vi "DataTreeCtrl signalToSpecData.vi"(8 "error in (no error)":errorcluster, 10 "signalMultiData":waveform(sgl)[](array[waveform]), 11 "DataTreeCtrl in":refnum<class "DataTreeCtrl.lvclass">) -> (0 "error out":errorcluster, 1 "labelName":T2, 2 "scanSigInfo":T1(array[cluster]), 3 "DataTreeCtrl out":refnum<class "DataTreeCtrl.lvclass">, 4 "mergeValid?":bool, 5 "plotName":string[](array[string]))   [LabVIEW 2018, in "DataTreeCtrl.lvclass"]
uses:
  DataTreeCtrl.lvclass
  DataTreeCtrl.lvclass/DataTreeCtrl.ctl
  PublicSubVI/Overload/Experiment Condition/_PC_Pub_ExpCondiValue_Script.vi
  PublicSubVI/Class/Sig2MS/Sig2MS.lvclass
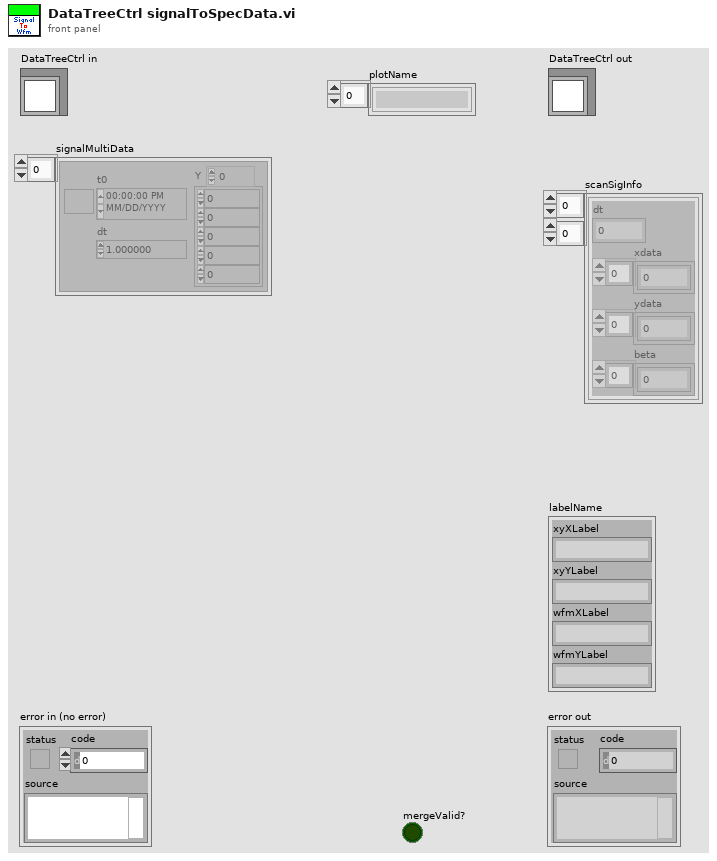
[diagram p1: front panel]
types:
  T1 = cluster{"dt":dbl, "xdata":dbl[], "ydata":sgl[], "beta":dbl[]}[][]
  T2 = cluster{"xyXLabel":string, "xyYLabel":string, "wfmXLabel":string, "wfmYLabel":string}
  T3 = enum16{"init", "loadScript", "newScript", "runScript", "close"}
  T4 = cluster{"startTime":dbl, "scanSig":cluster{"priDt":dbl, "priXData":dbl[], "priYData":sgl[], "beta":dbl[]}[], "ionSig":cluster{"secDt":dbl, "secYData":sgl[]}[]}
  T5 = cluster{"startTime":dbl, "scanData":cluster{"dt":dbl, "xdata":dbl[], "ydata":sgl[], "beta":dbl[]}[], "xyXLabel":string, "xyYLabel":string, "wfmXLabel":string, "wfmYLabel":string, "ionData":cluster{"dt":dbl, "ydata":sgl[]}[], "ionXLabel":string, "ionYLabel":string}
  T6 = cluster{"dt":dbl, "xdata":dbl[], "ydata":sgl[], "beta":dbl[]}[]
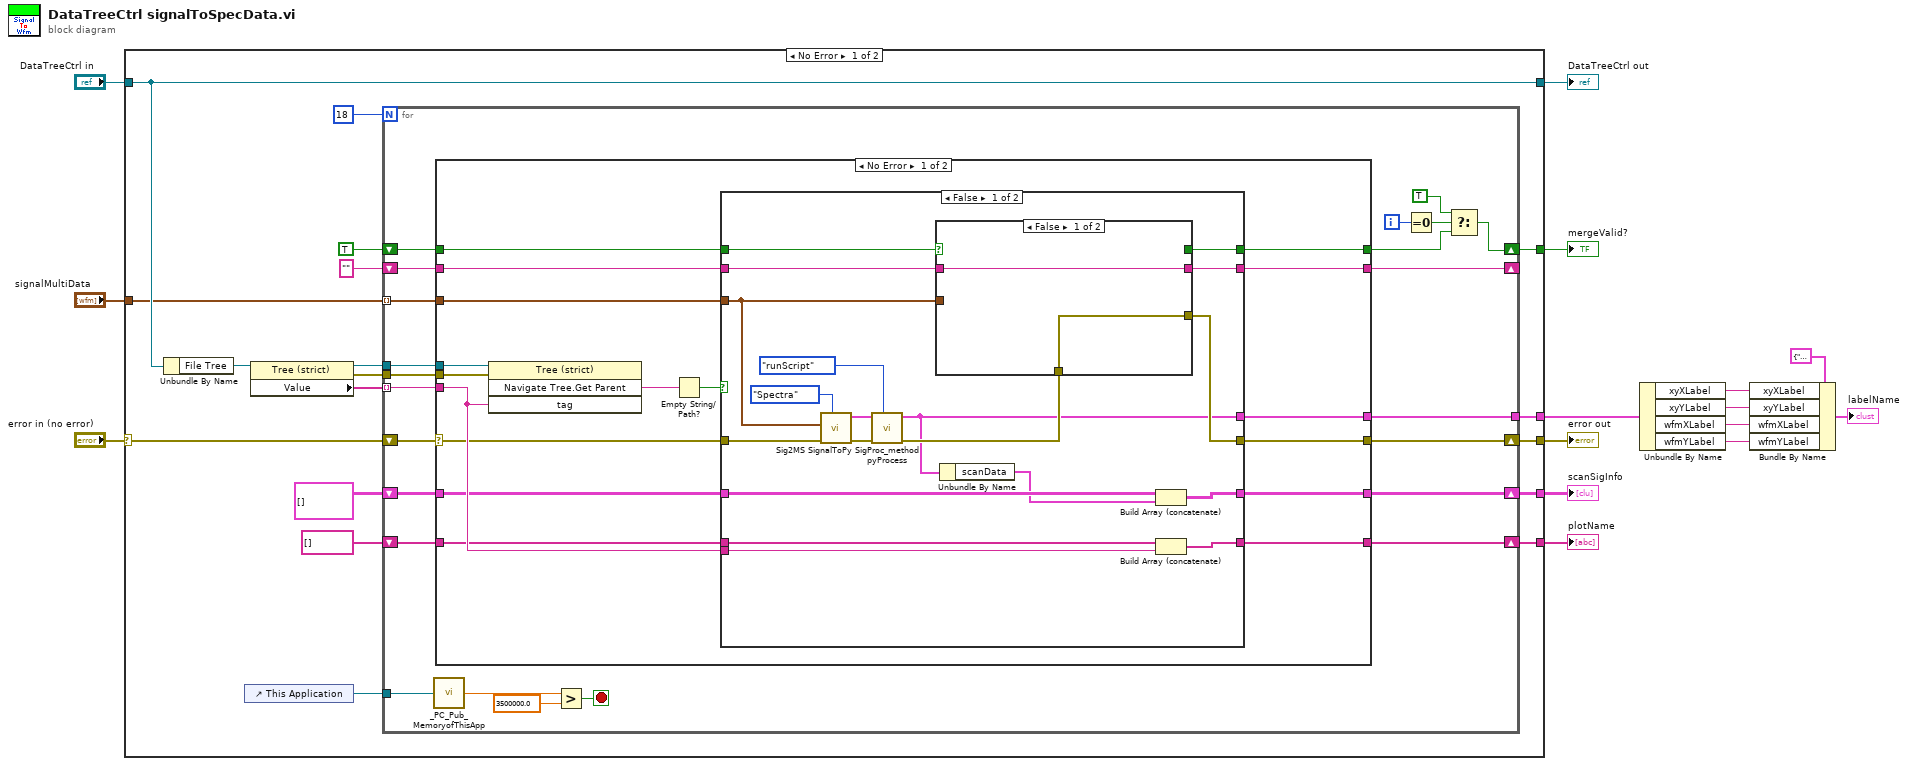
[diagram p0: block diagram]
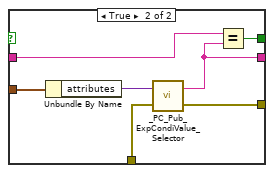
[diagram p2: hidden frame]
diagram:
  n1 = case shown="No Error" "error in (no error)" {
    selector: "error in (no error)" -> [w27 w113]
    tunnel: [w23 w113] -> w12
    tunnel: [w33 w112] -> w13
    tunnel: "DataTreeCtrl in" -> [w33 w112]
    tunnel: [w29 _] -> w1
    tunnel: [w22 _] -> w11
    tunnel: [w20 _] -> w10
    tunnel: "signalMultiData" -> [w19 _]
    tunnel: [w17 _] -> w8
    frame No Error {
      n2 = Unbundle By Name(w33) -> ("File Tree"=w32:refnum<vi>)
      n3 = control-ref of="This Application"() -> (w28:refnum<vi>)
      n4 = property class="Tree (strict)"(reference=w32) -> (reference out=w31:refnum<vi>, error out=w30:errorcluster, "Value"=w18:string[])  [unwired: 1 in]
      n5 = for {
        N: 18 -> [_]
        tunnel: w18 -> [w39] mode=indexing
        tunnel: w31 -> [w56]
        tunnel: w30 -> [w55]
        shift-right: [w54] -> w29
        shift-left: T1 [] -> [w34]
        tunnel: w28 -> [w51]
        shift-right: [w50] -> w23
        shift-left: w27 -> [w49]
        shift-right: [w48] -> _
        shift-left: "" ("scriptCode") -> [w47]
        shift-right: [w41] -> w22
        shift-left: TRUE -> [w46]
        shift-right: [w37] -> w20
        shift-left: string[] [] ("wfmData") -> [w38]
        tunnel: w19 -> [w36] mode=indexing
        tunnel: [w35] -> w17
        i -> [w45]
        stop <- w40 stop-if-true
        n6 = call "_PC_Pub_MemoryofThisApp.vi"("ThisApp Ref"=w51) -> ("number"=w52:dbl)
        n7 = case shown="No Error" w49 {
          selector: w49 -> [w66 w111]
          tunnel: w56 -> [w73 _]
          tunnel: w55 -> [w72 _]
          tunnel: w39 -> [w70 _]
          tunnel: w34 -> [w69 w110]
          tunnel: [w68 w110] -> w54
          tunnel: [w67 w111] -> w50
          tunnel: [w65 w108] -> w48
          tunnel: w47 -> [w64 w108]
          tunnel: [w63 w109] -> w43
          tunnel: w46 -> [w62 w109]
          tunnel: w38 -> [w61 w107]
          tunnel: [w60 w107] -> w37
          tunnel: w36 -> [w59 _]
          tunnel: [w58 _] -> w35
          frame No Error {
            n8 = invoke class="Tree (strict)" method="Navigate Tree.Get Parent"(reference=w73, error in=w72, "tag"=w70) -> ("Navigate Tree:Get Parent"=w57:string)  [unwired: 1 in, 3 out]
            n9 = Empty String/Path?(string/path=w57) -> (empty?=w71:bool)
            n10 = case shown="False" w71 {
              tunnel: w70 -> [w76 _]
              tunnel: w69 -> [w78 w106]
              tunnel: [w92 w106] -> w68
              tunnel: [w91 w103] -> w67
              tunnel: w66 -> [w81 w103]
              tunnel: [w89 w104] -> w65
              tunnel: w64 -> [w90 w104]
              tunnel: [w88 w105] -> w63
              tunnel: w62 -> [w87 w105]
              tunnel: w61 -> [w86 w102]
              tunnel: [w85 w102] -> w60
              tunnel: w59 -> [w80 _]
              tunnel: [w74 _] -> w58
              frame False {
                n11 = call "Sig2MS SignalToPy.vi"("getType"=enum16{"All", "Spectra", "Ionisation"}."Spectra", "error in (no error)"=w81, "rawSignal"=w80) -> ("error out"=w84:errorcluster, "pySigFormat"=w83:T4)  [unwired: 7 in]
                n12 = call "SigProc_method pyProcess.vi"("func"=T3."runScript", "error in (no error)"=w84, "dataParam"=w83) -> ("error out"=w79:errorcluster, "newSigInfo"=w74:T5)  [unwired: 5 in, 2 out]
                n13 = case shown="False" w87 {
                  tunnel: w80 -> [_ w101]
                  tunnel: w79 -> [w94 w99]
                  tunnel: [w94 w98] -> w91
                  tunnel: w90 -> [w93 w97]
                  tunnel: [w93 w96] -> w89
                  tunnel: [_ w95] -> w88
                  frame False {
                  }
                  frame True {
                    n14 = Unbundle By Name(w101) -> ("attributes"=w100:variant)
                    n15 = call-poly "_PC_Pub_ExpCondiValue_Selector.vi"("error in (no error)"=w99, "expCondiVariant"=w100) -> ("error out"=w98:errorcluster, "scriptCode"=w96:string)
                    n16 = Equal?(x=w97, y=w96) -> (x = y?=w95:bool)
                  }
                }
                n17 = Unbundle By Name(w74) -> ("scanData"=w75:T6)
                n18 = Build Array (concatenate)(w78, w75) -> (w92:T1)
                n19 = Build Array (concatenate)(w86, w76) -> (w85:string[])
              }
              frame True {
              }
            }
          }
          frame Error {
          }
        }
        n20 = Greater?(x=w52, y=sgl 3500000.0) -> (0:w40:bool)
        n21 = Equal To 0?(x=w45) -> (x = 0?=w44:bool)
        n22 = Select(t=TRUE, s=w44, f=w43) -> (s? t:f=w41:bool)
      }
    }
    frame Error {
    }
  }
  "error out" <- w12
  "DataTreeCtrl out" <- w13
  "mergeValid?" <- w11
  "plotName" <- w10
  "scanSigInfo" <- w1
  n23 = Unbundle By Name(w8) -> ("xyXLabel"=w6:string, "xyYLabel"=w5:string, "wfmXLabel"=w4:string, "wfmYLabel"=w3:string)
  n24 = Bundle By Name(cluster=T2 {"xyXLabel"="", "xyYLabel"="", "wfmXLabel"="", "wfmYLabel"=""}, "xyXLabel"=w6, "xyYLabel"=w5, "wfmXLabel"=w4, "wfmYLabel"=w3) -> (→"labelName":T2)
